vi "Demo_Andon get max ID.vi"(8 "error in (no error)":errorcluster, 10 "Station No.":string, 11 "Refnum in":T1) -> (0 "error out":errorcluster, 1 "TABLE NAME":string, 2 "ID MAX":i32, 3 "Refnum out":T1)   [LabVIEW 2017]
uses:
  <vilib>/addons/database/Connection.llb/Conn ObjectReference.ctl
  <vilib>/addons/database/Connection.llb/Conn Execute.vi
  <vilib>/addons/database/Recordset.llb/Rec Fetch Recordset Data (R).vi
  <vilib>/addons/database/Recordset.llb/Rec Destroy - Connection.vi
  <vilib>/addons/database/NI_Database_API.lvlib
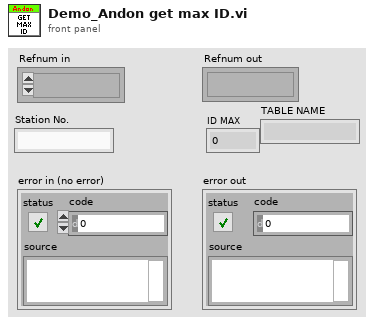
[diagram p1: front panel]
types:
  T1 = typedef "NI_Database_API.lvlib/Conn ObjectReference.ctl" = refnum<k1>
  T2 = typedef "NI_Database_API.lvlib/Rec ObjectReference.ctl" = refnum<k1>
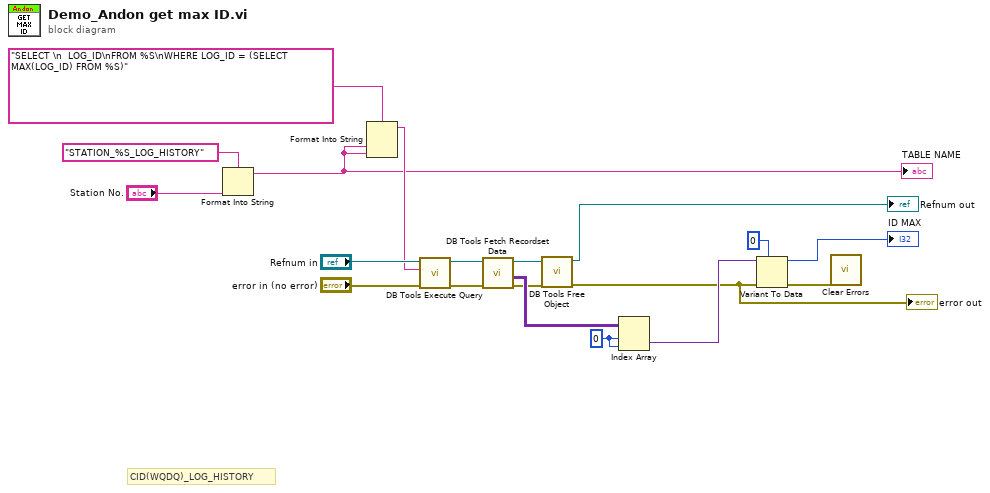
[diagram p0: block diagram]
diagram:
  w8 = 0 ("index (row)")
  # "CID(WQDQ)_LOG_HISTORY"
  n1 = Format Into String(format string="STATION_%S_LOG_HISTORY" ("SQL query"), "Station No.") -> (resulting string=w2:string)  [unwired: 2 in, 1 out]
  "TABLE NAME" <- w2
  n2 = Format Into String(format string="SELECT \n  LOG_ID\nFROM %S\nWHERE LOG_ID = (SELECT MAX(LOG_ID) FROM %S)" ("SQL query"), w2, w2) -> (resulting string=w6:string)  [unwired: 2 in, 1 out]
  n3 = call-poly <vilib>:"DB Tools Execute Query.vi"("error in (no error)"="error in (no error)", "SQL query"=w6, "connection reference"="Refnum in") -> ("error out"=w12:errorcluster, "recordset reference"=w13:T2)  [unwired: 5 in]
  n4 = call-poly <vilib>:"DB Tools Fetch Recordset Data.vi"("error in (no error)"=w12, "recordset reference"=w13) -> ("error out"=w11:errorcluster, "recordset data"=w15:variant[][], "recordset reference out"=w14:T2)  [unwired: 3 in]
  n5 = call-poly <vilib>:"DB Tools Free Object.vi"("error in (no error)"=w11, "recordset reference"=w14) -> ("error out"=w1:errorcluster, "connection reference"=→"Refnum out":T1)  [unwired: 8 in]
  "error out" <- w1
  n6 = Index Array(array=w15, index (row)=w8, index (col)=w8) -> (element=w9:variant)
  n7 = Variant To Data(error in=w1, type=0, Variant=w9) -> (data=→"ID MAX":i32, error out=w19:errorcluster)
  n8 = call <vilib>:"Clear Errors.vi"("error in (no error)"=w19) -> ()  [unwired: 5 in, 2 out]
